vi "Recipe example.vi"() -> ()   [LabVIEW 2020, in "SMCD14_lib.lvlib"]
uses:
  SMCD14_lib.lvlib
  Macro Cluster.ctl
  typedefAxisConfiguration.ctl
panel:
  in  "Actiomn":u16(ring) items=["NONE", "Start", "Stop", "Clear", "Motor ON", "Motor OFF"]
  in  "Move type:-NoCalib":u16(ring) items=["Absolute"=1, "Relative"=2, "Velocity"=3, "none"=0]
  in  "Move type:-Full":u16(ring) items=["Absolute"=1, "Relative"=2, "Velocity"=3, "Homing"=4, "none"=0]
  out "AllowCalib":bool
  in  "Recipe":i32(listbox)
  in  "Macro Cluster":T1={"Macro Type"=0, "Macro Name"="", "Macro Description"="", "M1_action_axis 1"=0, "M1_action_axis 2"=0, "M1_action_axis 3"=0, "M1_action_axis 4"=0, "M1_action_axis 5"=0, "M1_action_axis 6"=0, "M2_Axis"=0, "M2_Target_Pos"=0.0, "M2_Target_Vel"=0.0, "MoveModeControl"=0, "M3_1_Time"=0, "M3_Type"=0, "M3_2_wait_for_axis 1"=FALSE, "M3_2_wait_for_axis 2"=FALSE, "M3_2_wait_for_axis 3"=FALSE, "M3_2_wait_for_axis 4"=FALSE, "M3_2_wait_for_axis 5"=FALSE, "M3_2_wait_for_axis 6"=FALSE, "M3_3_mesage"="", "M3_3_wait_for_calib"=FALSE, "SelectedTargetCtrl"=1, "M5_select_action"=0} caption="Cluster 2" {"M5_select_action" items=["Stop", "Safe Position", "Working Position", "Run scaning", "Transfer posituin"]; "SelectedTargetCtrl" items=["none", "Target 1", "Target 2", "Target 3", "Target 4", "Target 5", "Target 6", "Laser test"]; "M3_Type" items=["Type1", "Type2", "Type3", "Type4", "Type5"]; "M3_1_Time" format="%<%H:%M:%S>t"; "MoveModeControl" items=["Absolute"=1, "Relative"=2, "Velocity"=3, "Homing"=4, "none"=0]; "M2_Target_Vel" format="%<%H:%M:%S>t"; "M2_Axis" items=["Axis no1", "Axis no2", "Axis no3", "Axis no4", "Axis no5", "Axis no6"]; "M1_action_axis 6" items=["NONE", "Start", "Stop", "Clear", "Motor ON", "motor OFF"]; "M1_action_axis 5" items=["NONE", "Start", "Stop", "Clear", "Motor ON", "motor OFF"]; "M1_action_axis 4" items=["NONE", "Start", "Stop", "Clear", "Motor ON", "motor OFF"]; "M1_action_axis 3" items=["------", "Manual", "Time SP", "Thickness SP"]; "M1_action_axis 2" items=["NONE", "Start", "Stop", "Clear", "Motor ON", "motor OFF"]; "M1_action_axis 1" items=["NONE", "Start", "Stop", "Clear", "Motor ON", "motor OFF"]; "Macro Type" items=["Action", "Parameters", "Wait"]}
  in  "Macro to add:":u16(ring) items=["Action", "Parameters", "Wait"]
  in  "Remove":bool
  in  "Add":bool
  in  "Next":bool
  in  "Back":bool
  out "AxisaMaxSpeed":dbl[](array[numeric])
  out "AxisaMinSpeed":dbl[](array[numeric])
  in  "AxisConfigurations":T2[](array[typedef]) {"AxisMaxSpeed" format="%#_6f"; "AxisMinSpeed" format="%#_6f"; "UnitsControl" items=["mm", "°"]}
  out "edit?":bool
  in  "Open Button":bool
  in  "Save Button":bool
  in  "New Button":bool
  in  "Macro Description:":string
  in  "Macro name:":string
  in  "Macro:":u16(ring) items=["Action", "Parameters", "Wait"]
  in  "Tab Control":enum32{"M1", "M2", "M3"}(tab)
  in  "Axis 1 action:":u16(ring) caption="Axis 1 axis action:" items=["NONE", "Start", "Stop", "Clear", "Motor ON", "Motor OFF"]
  in  "Axis 2 action:":u16(ring) caption="Axis 2 axis action:" items=["NONE", "Start", "Stop", "Clear", "Motor ON", "Motor OFF"]
  in  "Axis 3 action:":u16(ring) caption="Axis 2 axis action:" items=["NONE", "Start", "Stop", "Clear", "Motor ON", "Motor OFF"]
  in  "Axis 4 action:":u16(ring) caption="Axis 4 axis action:" items=["NONE", "Start", "Stop", "Clear", "Motor ON", "Motor OFF"]
  in  "Axis 5 action:":u16(ring) caption="Axis 5 axis action:" items=["NONE", "Start", "Stop", "Clear", "Motor ON", "Motor OFF"]
  in  "Axis 6 action:":u16(ring) caption="Axis 6 axis action:" items=["NONE", "Start", "Stop", "Clear", "Motor ON", "Motor OFF"]
  in  "Act. Step":i32
  in  "Axis:":u16(ring)
  in  "Target pos.:":sgl format="%#_6f unit"
  in  "Target vel.:":sgl caption="Wait Time" format="%#_6f unit/s"
  in  "Move type:":u16(ring) caption="Energy voltage SP:" items=["Absolute"=1, "Relative"=2, "Velocity"=3, "none"=0]
  in  "M3_Type":u16(ring) items=["Wait for time", "wait for axis", "wait for user action"]
  in  "Tab -Wait":enum32{"1", "2", "3"}(tab)
  in  "Time:":u32 caption="Shutter Time SP:" format="%<%H:%M:%S>t"
  out "Remaining\ntime:":i32 caption="Shutter Time SP:" format="%<%H:%M:%S>t"
  in  "wait for Homed":bool
  in  "wait for axis 1":bool
  in  "wait for axis 2":bool
  in  "wait for axis 3":bool
  in  "wait for axis 4":bool
  in  "wait for axis 5":bool
  in  "wait for axis 6":bool
  in  "Mesage:":string
  out "AxisNames":string[](array[string])
  in  "Current Macro":T1={"Macro Type"=0, "Macro Name"="", "Macro Description"="", "M1_action_axis 1"=0, "M1_action_axis 2"=0, "M1_action_axis 3"=0, "M1_action_axis 4"=0, "M1_action_axis 5"=0, "M1_action_axis 6"=0, "M2_Axis"=0, "M2_Target_Pos"=0.0, "M2_Target_Vel"=0.0, "MoveModeControl"=0, "M3_1_Time"=0, "M3_Type"=0, "M3_2_wait_for_axis 1"=FALSE, "M3_2_wait_for_axis 2"=FALSE, "M3_2_wait_for_axis 3"=FALSE, "M3_2_wait_for_axis 4"=FALSE, "M3_2_wait_for_axis 5"=FALSE, "M3_2_wait_for_axis 6"=FALSE, "M3_3_mesage"="", "M3_3_wait_for_calib"=FALSE, "SelectedTargetCtrl"=1, "M5_select_action"=0} caption="Cluster 2" {"M5_select_action" items=["Stop", "Safe Position", "Working Position", "Run scaning", "Transfer posituin"]; "SelectedTargetCtrl" items=["none", "Target 1", "Target 2", "Target 3", "Target 4", "Target 5", "Target 6", "Laser test"]; "M3_Type" items=["Type1", "Type2", "Type3", "Type4", "Type5"]; "M3_1_Time" format="%<%H:%M:%S>t"; "MoveModeControl" items=["Absolute"=1, "Relative"=2, "Velocity"=3, "Homing"=4, "none"=0]; "M2_Target_Vel" format="%<%H:%M:%S>t"; "M2_Axis" items=["Axis no1", "Axis no2", "Axis no3", "Axis no4", "Axis no5", "Axis no6"]; "M1_action_axis 6" items=["NONE", "Start", "Stop", "Clear", "Motor ON", "motor OFF"]; "M1_action_axis 5" items=["NONE", "Start", "Stop", "Clear", "Motor ON", "motor OFF"]; "M1_action_axis 4" items=["NONE", "Start", "Stop", "Clear", "Motor ON", "motor OFF"]; "M1_action_axis 3" items=["------", "Manual", "Time SP", "Thickness SP"]; "M1_action_axis 2" items=["NONE", "Start", "Stop", "Clear", "Motor ON", "motor OFF"]; "M1_action_axis 1" items=["NONE", "Start", "Stop", "Clear", "Motor ON", "motor OFF"]; "Macro Type" items=["Action", "Parameters", "Wait"]}
  in  "Macro Table":T1[](array[typedef]) {"M5_select_action" items=["Stop", "Safe Position", "Working Position", "Run scaning", "Transfer posituin"]; "SelectedTargetCtrl" items=["none", "Target 1", "Target 2", "Target 3", "Target 4", "Target 5", "Target 6", "Laser test"]; "M3_Type" items=["Type1", "Type2", "Type3", "Type4", "Type5"]; "M3_1_Time" format="%<%H:%M:%S>t"; "MoveModeControl" items=["Absolute"=1, "Relative"=2, "Velocity"=3, "Homing"=4, "none"=0]; "M2_Target_Vel" format="%<%H:%M:%S>t"; "M2_Axis" items=["Axis no1", "Axis no2", "Axis no3", "Axis no4", "Axis no5", "Axis no6"]; "M1_action_axis 6" items=["NONE", "Start", "Stop", "Clear", "Motor ON", "motor OFF"]; "M1_action_axis 5" items=["NONE", "Start", "Stop", "Clear", "Motor ON", "motor OFF"]; "M1_action_axis 4" items=["NONE", "Start", "Stop", "Clear", "Motor ON", "motor OFF"]; "M1_action_axis 3" items=["------", "Manual", "Time SP", "Thickness SP"]; "M1_action_axis 2" items=["NONE", "Start", "Stop", "Clear", "Motor ON", "motor OFF"]; "M1_action_axis 1" items=["NONE", "Start", "Stop", "Clear", "Motor ON", "motor OFF"]; "Macro Type" items=["Action", "Parameters", "Wait"]}
  out "size":i32
  # "Przykładowy silnik do zaawansowanych receptur w LabView\nw zależności od wybranego typu ukruwane/ pokazywane są \npola do edycji.\nw liście Recipe pokazywany jest podląd wszystkich receptur, \nmożna kliknąć w wybraną - okno Macro przełączy sie na wybraną\nnawigować moża przyciskami <-- i -->\nmożda dodać kolejne makro lub usunąc aktywne"
  # "Lista makr:\nx- SET data:\nx    Power SP\nx    Voltage SP\nx    Current SP\n\nx- SET shutter data\nx    Working mode - Manual nie dostępny\nx    Thicknes SP\nx    Time SP\n\nx- SET MFC setpoint\nx    Flow SP\n\nx- SET Operate/Standby\nx- Open/Close Shutter\nx- Open/Close MFC\n- Wait for Time\n    Time \n- wait for close Shutter"
  # "Select action for each axes:"
  # "Set axis parameters:"
  # "Select wait mode:"
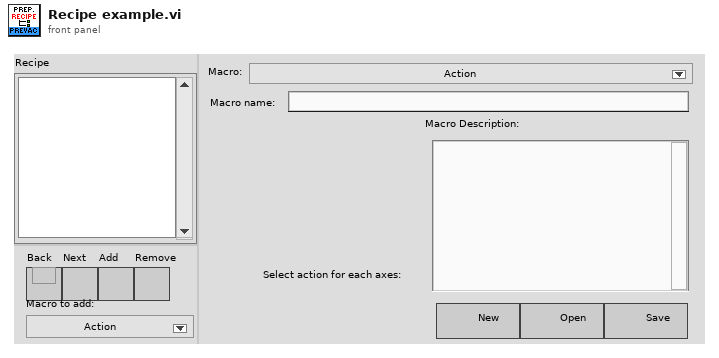
[diagram p1: front panel]
types:
  T1 = typedef "SMCD14_lib.lvlib/Macro Cluster.ctl" = cluster{"Macro Type":u16, "Macro Name":string, "Macro Description":string, "M1_action_axis 1":u16, "M1_action_axis 2":u16, "M1_action_axis 3":u16, "M1_action_axis 4":u16, "M1_action_axis 5":u16, "M1_action_axis 6":u16, "M2_Axis":u16, "M2_Target_Pos":sgl, "M2_Target_Vel":sgl, "MoveModeControl":u16, "M3_1_Time":u32, "M3_Type":u16, "M3_2_wait_for_axis 1":bool, "M3_2_wait_for_axis 2":bool, "M3_2_wait_for_axis 3":bool, "M3_2_wait_for_axis 4":bool, "M3_2_wait_for_axis 5":bool, "M3_2_wait_for_axis 6":bool, "M3_3_mesage":string, "M3_3_wait_for_calib":bool, "SelectedTargetCtrl":u16, "M5_select_action":u16}
  T2 = typedef "SMCD14_lib.lvlib/typedefAxisConfiguration.ctl" = cluster{"AxisName":string, "UnitsControl":u16, "AxisSlaveID":u16, "AxisBaseAddr":u16, "AxisMinSpeed":dbl, "AxisMaxSpeed":dbl}
  T3 = enum16{"open", "replace", "create", "open or create", "replace or create", "replace or create with confirmation"}
  T4 = typedef "LVStringsAndValuesArrayTypeDef_U16.ctl" = cluster{"String":string, "Value":u16}[]
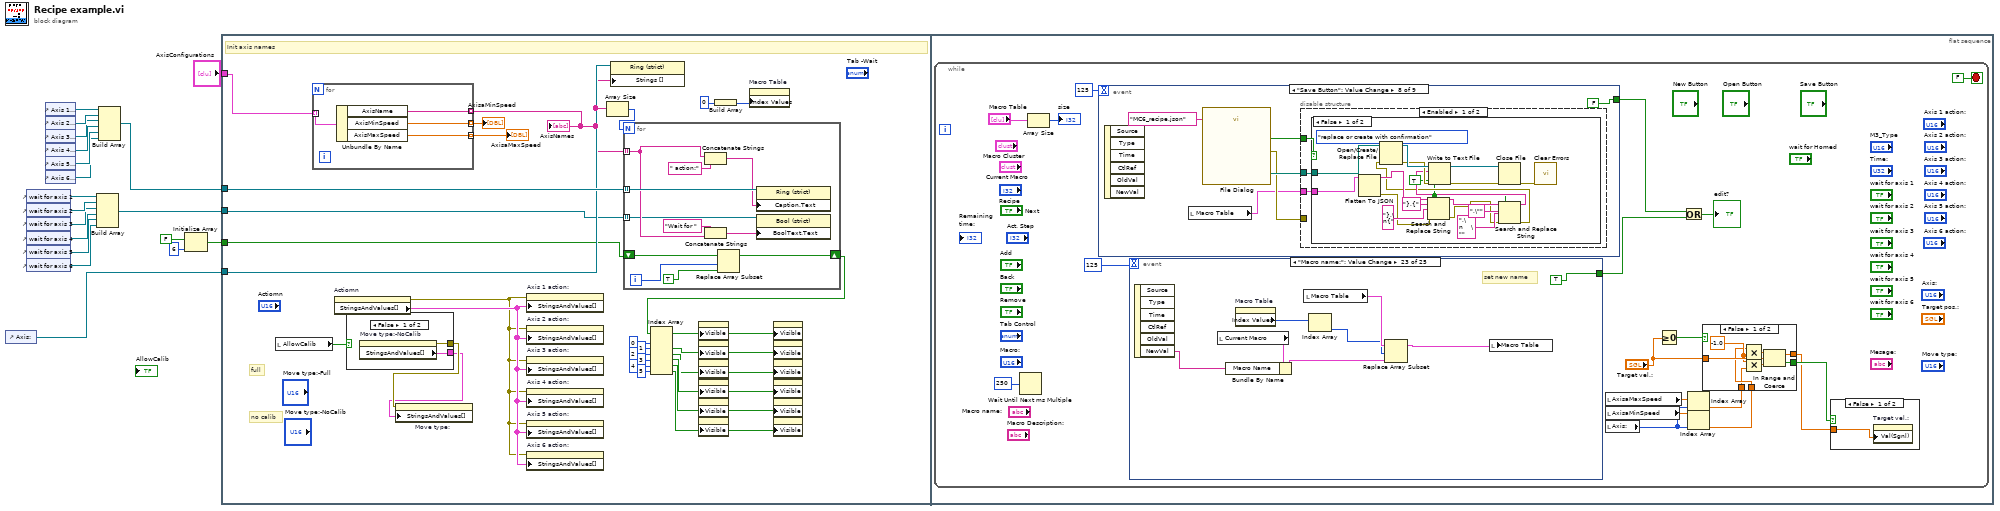
[diagram p0: block diagram]
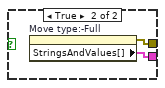
[diagram p2: hidden frame]
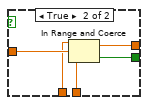
[diagram p4: hidden frame]
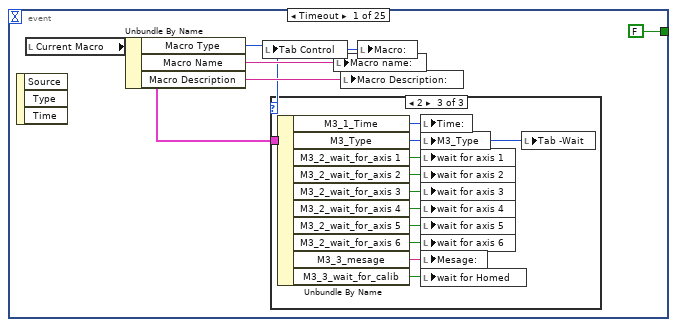
[diagram p5: hidden frame]
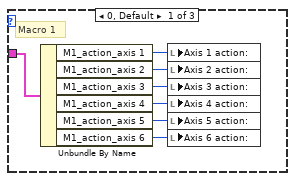
[diagram p6: hidden frame]
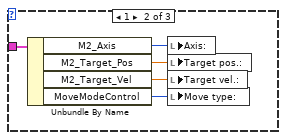
[diagram p7: hidden frame]
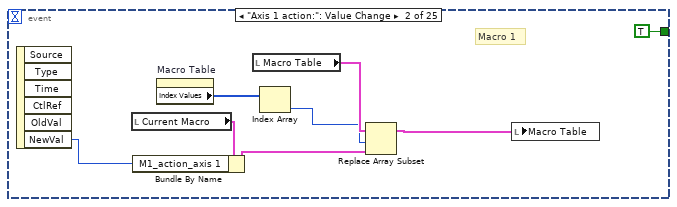
[diagram p8: hidden frame]
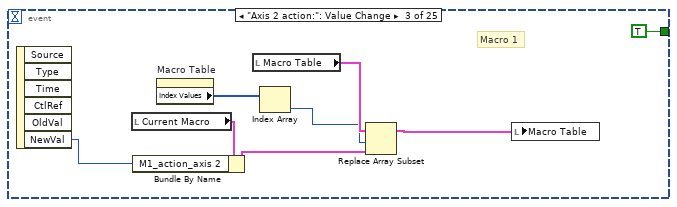
[diagram p9: hidden frame]
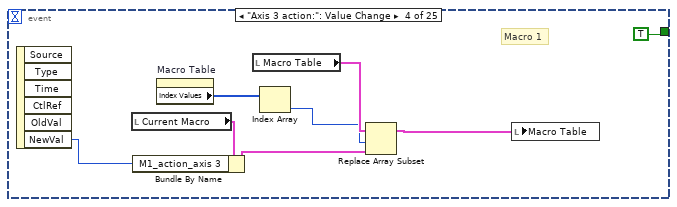
[diagram p10: hidden frame]
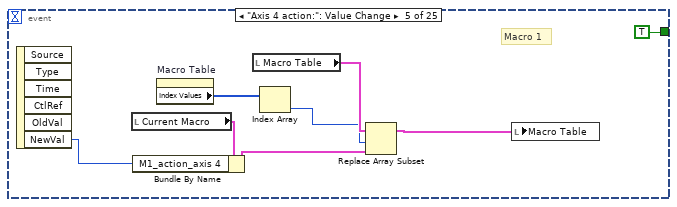
[diagram p11: hidden frame]
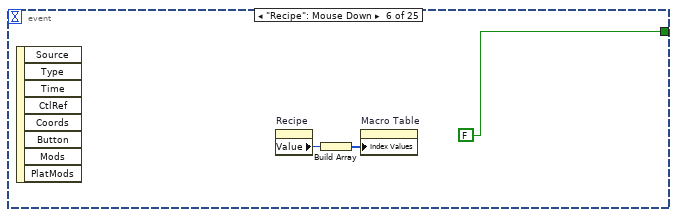
[diagram p12: hidden frame]
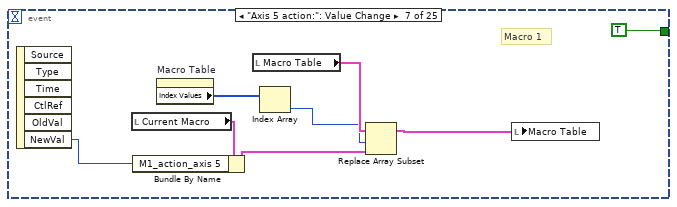
[diagram p13: hidden frame]
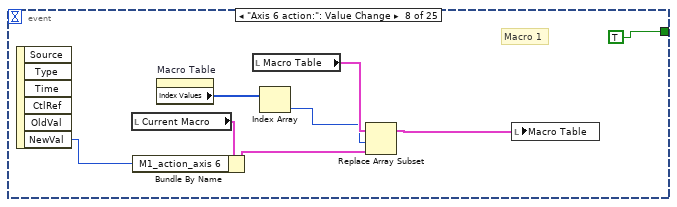
[diagram p14: hidden frame]
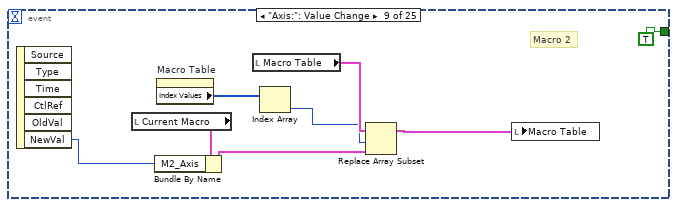
[diagram p15: hidden frame]
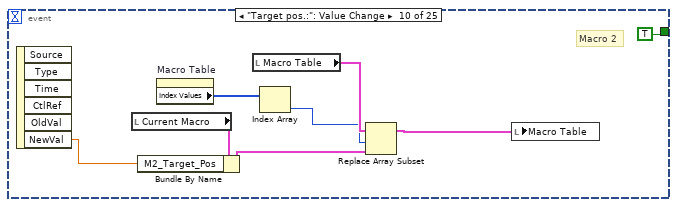
[diagram p16: hidden frame]
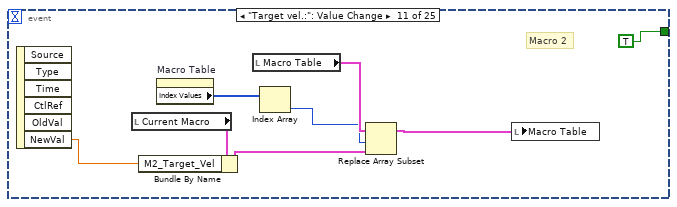
[diagram p17: hidden frame]
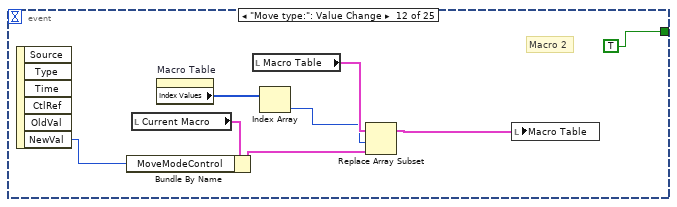
[diagram p18: hidden frame]
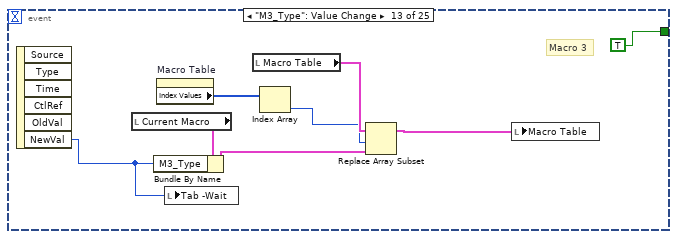
[diagram p19: hidden frame]
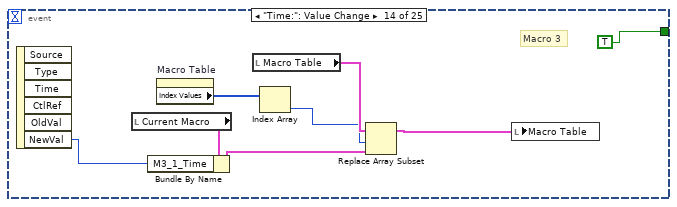
[diagram p20: hidden frame]
diagram:
  n1 = control-ref of="Axis:"() -> (w12:refnum<vi>)
  n2 = control-ref of="wait for axis 1"() -> (w11:refnum<vi>)
  n3 = control-ref of="wait for axis 2"() -> (w10:refnum<vi>)
  n4 = control-ref of="wait for axis 3"() -> (w9:refnum<vi>)
  n5 = control-ref of="wait for axis 4"() -> (w6:refnum<vi>)
  n6 = control-ref of="wait for axis 5"() -> (w8:refnum<vi>)
  n7 = control-ref of="wait for axis 6"() -> (w7:refnum<vi>)
  n8 = control-ref of="Axis 1 action:"() -> (w19:refnum<vi>)
  n9 = control-ref of="Axis 2 action:"() -> (w14:refnum<vi>)
  n10 = control-ref of="Axis 3 action:"() -> (w13:refnum<vi>)
  n11 = control-ref of="Axis 4 action:"() -> (w18:refnum<vi>)
  n12 = control-ref of="Axis 5 action:"() -> (w17:refnum<vi>)
  n13 = control-ref of="Axis 6 action:"() -> (w16:refnum<vi>)
  n14 = Build Array(w11, w10, w9, w6, w8, w7) -> (w5:refnum<vi>[])
  n15 = Build Array(w19, w14, w13, w18, w17, w16) -> (w15:refnum<vi>[])
  n16 = Initialize Array(FALSE, 6 ("dimension size")) -> (w1:bool[])
  n17 = flat-sequence {
    tunnel: w15 -> [w48]
    tunnel: w12 -> [w47]
    tunnel: w5 -> [w46]
    tunnel: "AxisConfigurations" -> [w44]
    tunnel: w1 -> [w36]
    frame #0 {
      # "no calib"
      # "full"
      # "Init axis names"
      n18 = local read "AllowCalib"() -> (w41:bool)
      n19 = for {
        tunnel: w44 -> [w56] mode=indexing
        tunnel: [w55] -> w28 mode=indexing
        tunnel: [w54] -> w43 mode=indexing
        tunnel: [w53] -> w42 mode=indexing
        n20 = Unbundle By Name(w56) -> ("AxisName"=w55:string, "AxisMinSpeed"=w54:dbl, "AxisMaxSpeed"=w53:dbl)
      }
      "AxisNames" <- w28
      "AxisaMinSpeed" <- w43
      "AxisaMaxSpeed" <- w42
      n21 = property on="Actiomn" class="Ring (strict)"() -> (error out=w39:errorcluster, "StringsAndValues[]"=w40:T4)  [unwired: 2 in, 1 out]
      n22 = case shown="False" w41 {
        tunnel: [w50 w51] -> w37
        tunnel: [w49 w52] -> w38
        frame False {
          n23 = property on="Move type:-NoCalib" class="Ring (strict)"() -> (error out=w49:errorcluster, "StringsAndValues[]"=w50:T4)  [unwired: 2 in, 1 out]
        }
        frame True {
          n24 = property on="Move type:-Full" class="Ring (strict)"() -> (error out=w52:errorcluster, "StringsAndValues[]"=w51:T4)  [unwired: 2 in, 1 out]
        }
      }
      n25 = property on="Move type:" class="Ring (strict)"(error in=w38, "StringsAndValues[]"=w37) -> ()  [unwired: 1 in, 2 out]
      n26 = property on="Axis 1 action:" class="Ring (strict)"(error in=w39, "StringsAndValues[]"=w40) -> ()  [unwired: 1 in, 2 out]
      n27 = property on="Axis 2 action:" class="Ring (strict)"(error in=w39, "StringsAndValues[]"=w40) -> ()  [unwired: 1 in, 2 out]
      n28 = property on="Axis 3 action:" class="Ring (strict)"(error in=w39, "StringsAndValues[]"=w40) -> ()  [unwired: 1 in, 2 out]
      n29 = property on="Axis 4 action:" class="Ring (strict)"(error in=w39, "StringsAndValues[]"=w40) -> ()  [unwired: 1 in, 2 out]
      n30 = property on="Axis 5 action:" class="Ring (strict)"(error in=w39, "StringsAndValues[]"=w40) -> ()  [unwired: 1 in, 2 out]
      n31 = property on="Axis 6 action:" class="Ring (strict)"(error in=w39, "StringsAndValues[]"=w40) -> ()  [unwired: 1 in, 2 out]
      n32 = Array Size(array=w28) -> (size(s)=w27:i32)
      n33 = property class="Ring (strict)"(reference=w47, "Strings []"=w28) -> ()  [unwired: 1 in, 2 out]
      n34 = for {
        N: w27 -> [_]
        tunnel: w28 -> [w63] mode=indexing
        tunnel: w48 -> [w66] mode=indexing
        tunnel: w46 -> [w61] mode=indexing
        shift-right: [w57] -> w29
        shift-left: w36 -> [w60]
        i -> [w59]
        n35 = Concatenate Strings(w63, " action:" ("Label.Text")) -> (w65:string)
        n36 = Concatenate Strings("Wait for " ("Label.Text"), w63) -> (w62:string)
        n37 = Replace Array Subset(array=w60, new element=TRUE, index=w59) -> (w57:bool[])
        n38 = property class="Ring (strict)"(reference=w66, "Caption.Text"=w65) -> ()  [unwired: 1 in, 2 out]
        n39 = property class="Bool (strict)"(reference=w61, "BoolText.Text"=w62) -> ()  [unwired: 1 in, 2 out]
      }
      n40 = Index Array(array=w29, index #1=0 ("dimension size"), index #2=1 ("dimension size"), index #3=2 ("dimension size"), index #4=3 ("dimension size"), index #5=4 ("dimension size"), index #6=5 ("dimension size")) -> (element #1=w26:bool, element #2=w25:bool, element #3=w21:bool, element #4=w24:bool, element #5=w23:bool, element #6=w22:bool)
      n41 = property on="Axis 1 action:" class="Ring (strict)"("Visible"=w26) -> ()  [unwired: 2 in, 2 out]
      n42 = property on="Axis 2 action:" class="Ring (strict)"("Visible"=w25) -> ()  [unwired: 2 in, 2 out]
      n43 = property on="Axis 3 action:" class="Ring (strict)"("Visible"=w21) -> ()  [unwired: 2 in, 2 out]
      n44 = property on="Axis 4 action:" class="Ring (strict)"("Visible"=w24) -> ()  [unwired: 2 in, 2 out]
      n45 = property on="Axis 5 action:" class="Ring (strict)"("Visible"=w23) -> ()  [unwired: 2 in, 2 out]
      n46 = property on="Axis 6 action:" class="Ring (strict)"("Visible"=w22) -> ()  [unwired: 2 in, 2 out]
      n47 = Build Array(0) -> (w20:i32[])
      n48 = property on="Macro Table" class="Arr (strict)"("Index Values"=w20) -> ()  [unwired: 2 in, 2 out]
      n49 = property on="wait for axis 1" class="Bool (strict)"("Visible"=w26) -> ()  [unwired: 2 in, 2 out]
      n50 = property on="wait for axis 2" class="Bool (strict)"("Visible"=w25) -> ()  [unwired: 2 in, 2 out]
      n51 = property on="wait for axis 3" class="Bool (strict)"("Visible"=w21) -> ()  [unwired: 2 in, 2 out]
      n52 = property on="wait for axis 4" class="Bool (strict)"("Visible"=w24) -> ()  [unwired: 2 in, 2 out]
      n53 = property on="wait for axis 5" class="Bool (strict)"("Visible"=w23) -> ()  [unwired: 2 in, 2 out]
      n54 = property on="wait for axis 6" class="Bool (strict)"("Visible"=w22) -> ()  [unwired: 2 in, 2 out]
    }
    frame #1 {
      n55 = while {
        stop <- FALSE ("stop") stop-if-true
        n56 = Wait Until Next ms Multiple(millisecond multiple=u32 250) -> ()  [unwired: 1 out]
        n57 = Array Size(array="Macro Table") -> (size(s)=→"size":i32)
        n58 = event shown="[7] \"Save Button\": Value Change" {
          selector: _ -> [_ _ _ _ _ _ _ _ _]
          dyn-events: _ -> [_ _ _ _ _ _ _ _ _]
          timeout: 125 -> [_ _ _ _ _ _ _ _ _]
          tunnel: [FALSE FALSE FALSE FALSE TRUE TRUE TRUE FALSE TRUE] -> w79
          event Timeout {
            n59 = event-data() -> ()  [unwired: 1 in, 3 out]
            n60 = local read "Macro Table"() -> (w319:T1[])
            n61 = property on="Macro Table" class="Arr (strict)"() -> ("Index Values"=w321:u32[])  [unwired: 2 in, 2 out]
            n62 = for {
              tunnel: w319 -> [w333] mode=indexing
              tunnel: [w329] -> w317 mode=indexing
              tunnel: [w322] -> w316 mode=indexing
              i -> [w325]
              n63 = local read "Act. Step"() -> (w324:i32)
              n64 = Unbundle By Name(w333) -> ("Macro Type"=w331:u16, "Macro Name"=w326:string)
              n65 = property on="Macro to add:" class="Ring (strict)"() -> ("Strings []"=w332:string[])  [unwired: 2 in, 2 out]
              n66 = Subtract(x=w325, y=w324) -> (x-y=w323:i32)
              n67 = Index Array(array=w332, index=w331) -> (element=w330:string)
              n68 = case shown="..-1, Default" w323 {
                tunnel: [1 4 0] -> w322
                frame ..-1, Default {
                }
                frame 0 {
                }
                frame 1.. {
                }
              }
              n69 = Concatenate Strings(w330, "\r", "   | ", w326) -> (w329:string)
            }
            n70 = Index Array(array=w321) -> (element=w320:u32)  [unwired: 1 in]
            n71 = local write "Recipe"(w320) -> ()
            n72 = Index Array(array=w319, index=w320) -> (element=w318:T1)
            n73 = local write "Current Macro"(w318) -> ()
            n74 = property on="Recipe" class="LstBox (strict)"("Item Names"=w317) -> ()  [unwired: 2 in, 2 out]
            n75 = property on="Recipe" class="LstBox (strict)"("Item Symbols"=w316) -> ()  [unwired: 2 in, 2 out]
          }
          event Panel Close {
            n76 = event-data() -> ()  [unwired: 1 in, 4 out]
            n77 = Stop(stop? (T)=TRUE) -> ()
          }
          event "Next": Value Change {
            n78 = event-data() -> ()  [unwired: 1 in, 6 out]
            n79 = property on="Macro Table" class="Arr (strict)"() -> ("Index Values"=w340:u32[])  [unwired: 2 in, 2 out]
            n80 = local read "size"() -> (w345:i32)
            n81 = Index Array(array=w340) -> (element=w343:u32)  [unwired: 1 in]
            n82 = Decrement(x=w345) -> (x-1=w344:i32)
            n83 = Increment(x=w343) -> (x+1=w346:u32)
            n84 = In Range and Coerce(upper limit=w344, x=w346, lower limit=i16 0) -> (coerced(x)=w342:u32)  [unwired: 1 out]
            n85 = Build Array(w342) -> (w341:u32[])
            n86 = property on="Macro Table" class="Arr (strict)"("Index Values"=w341) -> ()  [unwired: 2 in, 2 out]
          }
          event "Back": Value Change {
            n87 = event-data() -> ()  [unwired: 1 in, 6 out]
            n88 = property on="Macro Table" class="Arr (strict)"() -> ("Index Values"=w352:u32[])  [unwired: 2 in, 2 out]
            n89 = Index Array(array=w352) -> (element=w351:u32)  [unwired: 1 in]
            n90 = Less Or Equal To 0?(x=w351) -> (x <= 0?=w353:bool)
            n91 = case shown="False" w353 {
              tunnel: w351 -> [w355 w356]
              tunnel: [w354 w356] -> w350
              frame False {
                n92 = Decrement(x=w355) -> (x-1=w354:u32)
              }
              frame True {
              }
            }
            n93 = Build Array(w350) -> (w349:u32[])
            n94 = property on="Macro Table" class="Arr (strict)"("Index Values"=w349) -> ()  [unwired: 2 in, 2 out]
          }
          event "Remove": Value Change {
            n95 = event-data() -> ()  [unwired: 1 in, 6 out]
            n96 = local read "size"() -> (w358:i32)
            n97 = property on="Macro Table" class="Arr (strict)"() -> ("Index Values"=w362:u32[])  [unwired: 2 in, 2 out]
            n98 = Index Array(array=w362) -> (element=w361:u32)  [unwired: 1 in]
            n99 = Greater?(x=w358, y=u32 1) -> (0:w359:bool)
            n100 = case shown="True" w359 {
              tunnel: w361 -> [_ w365]
              frame False {
              }
              frame True {
                n101 = local read "Macro Table"() -> (w367:T1[])
                n102 = Decrement(x=w365) -> (x-1=w364:u32)
                n103 = Delete From Array(array=w367, index=w365) -> (array with subset deleted=w366:T1[])  [unwired: 1 in, 1 out]
                n104 = local write "Macro Table"(w366) -> ()
                n105 = Build Array(w364) -> (w363:u32[])
                n106 = property on="Macro Table" class="Arr (strict)"("Index Values"=w363) -> ()  [unwired: 2 in, 2 out]
              }
            }
          }
          event "Add": Value Change {
            n107 = event-data() -> ()  [unwired: 1 in, 6 out]
            n108 = property on="Macro Table" class="Arr (strict)"() -> ("Index Values"=w377:u32[])  [unwired: 2 in, 2 out]
            n109 = local read "Macro Cluster"() -> (w370:T1)
            n110 = local read "Macro Table"() -> (w375:T1[])
            n111 = Bundle By Name(cluster=w370, "Macro Type"="Macro to add:") -> (w369:T1)
            n112 = Index Array(array=w377) -> (element=w374:u32)  [unwired: 1 in]
            n113 = Increment(x=w374) -> (x+1=w372:u32)
            n114 = Insert Into Array(array=w375, index=w372, new element=w369) -> (w373:T1[])
            n115 = Build Array(w372) -> (w376:u32[])
            n116 = local write "Macro Table"(w373) -> ()
            n117 = property on="Macro Table" class="Arr (strict)"("Index Values"=w376) -> ()  [unwired: 2 in, 2 out]
          }
          event "New Button": Value Change {
            n118 = event-data() -> ()  [unwired: 1 in, 6 out]
            n119 = Build Array(0) -> (w380:i32[])
            n120 = property on="Macro Table" class="Arr (strict)"("Index Values"=w380) -> ()  [unwired: 2 in, 2 out]
            n121 = local write "Macro Table"(T1[] [{"Macro Type"=0, "Macro Name"="", "Macro Description"="", "M1_action_axis 1"=0, "M1_action_axis 2"=0, "M1_action_axis 3"=0, "M1_action_axis 4"=0, "M1_action_axis 5"=0, "M1_action_axis 6"=0, "M2_Axis"=0, "M2_Target_Pos"=0.0, "M2_Target_Vel"=0.0, "MoveModeControl"=0, "M3_1_Time"=0, "M3_Type"=0, "M3_2_wait_for_axis 1"=FALSE, "M3_2_wait_for_axis 2"=FALSE, "M3_2_wait_for_axis 3"=FALSE, "M3_2_wait_for_axis 4"=FALSE, "M3_2_wait_for_axis 5"=FALSE, "M3_2_wait_for_axis 6"=FALSE, "M3_3_mesage"="", "M3_3_wait_for_calib"=FALSE, "SelectedTargetCtrl"=1, "M5_select_action"=0}] ("Macro Table")) -> ()
          }
          event "Save Button": Value Change {
            n122 = event-data() -> ()  [unwired: 1 in, 6 out]
            n123 = local read "Macro Table"() -> (w382:T1[])
            n124 = call "File Dialog"("default name"="MC6_recipe.json") -> ("selected path"=w385:path, "cancelled"=w386:bool, "error out"=w383:errorcluster)  [unwired: 11 in, 1 out]
            n125 = disable-structure shown="Enabled" {
              disable-tunnel: w386 -> [w390 w413]
              disable-tunnel: w385 -> [w389 w412]
              disable-tunnel: w382 -> [w388 w411]
              disable-tunnel: w383 -> [_ w410]
              frame Enabled {
                n126 = case shown="False" w390 {
                  tunnel: w389 -> [w409 _]
                  tunnel: w388 -> [w402 _]
                  frame False {
                    w391 = TRUE ("replace all? (F)")
                    n127 = Flatten To JSON(anything=w402) -> (JSON string=w398:string, 11:w399:errorcluster)  [unwired: 2 in]
                    n128 = Search and Replace String(replace all?=w391, input string=w398, search string="},{", replace string="},\n{" ("search string"), error in=w399) -> (result string=w397:string, error out=w393:errorcluster)  [unwired: 3 in, 2 out]
                    n129 = Search and Replace String(replace all?=w391, input string=w397, search string=",\"", replace string=",\n    \"" ("search string"), error in=w393) -> (result string=w394:string, error out=w392:errorcluster)  [unwired: 3 in, 2 out]
                    n130 = Open/Create/Replace File(file path (use dialog)=w409, error in=w392, operation (0:open)=T3."replace or create with confirmation") -> (refnum out=w407:refnum<file>, error out=w406:errorcluster)  [unwired: 3 in, 1 out]
                    n131 = Write to Text File(file (use dialog)=w407, text=w394, error in=w406) -> (refnum out=w405:refnum<file>, error out=w404:errorcluster)  [unwired: 1 in, 1 out]
                    n132 = Close File(refnum=w405, error in=w404) -> (error out=w403:errorcluster)  [unwired: 1 out]
                    n133 = call <vilib>:"Clear Errors.vi"("error in (no error)"=w403) -> ()  [unwired: 5 in, 2 out]
                  }
                  frame True {
                  }
                }
              }
              frame Disabled {
                n134 = case shown="False" w413 {
                  tunnel: w412 -> [w423 _]
                  tunnel: w411 -> [w416 _]
                  tunnel: w410 -> [w415 _]
                  frame False {
                    (unwired) TRUE ("replace all? (F)")
                    n135 = Flatten To XML(6:w416) -> (2:w414:string)
                    n136 = Open/Create/Replace File(file path (use dialog)=w423, error in=w415, operation (0:open)=T3."replace or create with confirmation") -> (refnum out=w421:refnum<file>, error out=w420:errorcluster)  [unwired: 3 in, 1 out]
                    n137 = Write to Text File(file (use dialog)=w421, text=w414, error in=w420) -> (refnum out=w419:refnum<file>, error out=w418:errorcluster)  [unwired: 1 in, 1 out]
                    n138 = Close File(refnum=w419, error in=w418) -> (error out=w417:errorcluster)  [unwired: 1 out]
                    n139 = call <vilib>:"Clear Errors.vi"("error in (no error)"=w417) -> ()  [unwired: 5 in, 2 out]
                  }
                  frame True {
                  }
                }
              }
            }
          }
          event "Open Button": Value Change {
            n140 = event-data() -> ()  [unwired: 1 in, 6 out]
            n141 = local read "Macro Table"() -> (w427:T1[])
            n142 = call "File Dialog2"("default name"="MC6_recipe.json") -> ("selected path"=w429:path, "exists"=w428:bool, "cancelled"=w430:bool)  [unwired: 11 in, 1 out]
            n143 = case shown="False" w430 {
              tunnel: w429 -> [w435 _]
              tunnel: w428 -> [w433 _]
              tunnel: w427 -> [w434 _]
              tunnel: [w432 0] -> w425
              frame False {
                n144 = disable-structure shown="Enabled" {
                  disable-tunnel: w435 -> [w439 w452]
                  disable-tunnel: w434 -> [w438 w451]
                  disable-tunnel: w433 -> [w437 w453]
                  disable-tunnel: [0 _] -> w432
                  frame Enabled {
                    n145 = case shown="True" w437 {
                      tunnel: w439 -> [_ w450]
                      tunnel: w438 -> [_ w444]
                      frame False {
                      }
                      frame True {
                        n146 = Open/Create/Replace File(file path (use dialog)=w450, operation (0:open)=T3."open") -> (refnum out=w447:refnum<file>, error out=w446:errorcluster)  [unwired: 4 in, 1 out]
                        n147 = Read from Text File(file (use dialog)=w447, error in=w446) -> (refnum out=w440:refnum<file>, text=w445:string, error out=w441:errorcluster)  [unwired: 2 in, 1 out]
                        n148 = Unflatten From JSON(JSON string=w445, type and defaults=w444, error in (no error)=w441) -> (value=w443:T1[], error out=w442:errorcluster)  [unwired: 4 in]
                        n149 = Close File(refnum=w440, error in=w442) -> (error out=w448:errorcluster)  [unwired: 1 out]
                        n150 = local write "Macro Table"(w443) -> ()
                        n151 = call <vilib>:"Clear Errors.vi"("error in (no error)"=w448) -> ()  [unwired: 5 in, 2 out]
                      }
                    }
                  }
                  frame Disabled {
                    n152 = case shown="True" w453 {
                      tunnel: w452 -> [_ w464]
                      tunnel: w451 -> [_ w458]
                      frame False {
                      }
                      frame True {
                        n153 = Open/Create/Replace File(file path (use dialog)=w464, operation (0:open)=T3."open") -> (refnum out=w461:refnum<file>, error out=w460:errorcluster)  [unwired: 4 in, 1 out]
                        n154 = Read from Text File(file (use dialog)=w461, error in=w460) -> (refnum out=w459:refnum<file>, text=w457:string, error out=w456:errorcluster)  [unwired: 2 in, 1 out]
                        n155 = Unflatten From XML(xml string=w457, type=w458, error in (no error)=w456) -> (value=w455:T1[], error out=w454:errorcluster)
                        n156 = Close File(refnum=w459, error in=w454) -> (error out=w462:errorcluster)  [unwired: 1 out]
                        n157 = local write "Macro Table"(w455) -> ()
                        n158 = call <vilib>:"Clear Errors.vi"("error in (no error)"=w462) -> ()  [unwired: 5 in, 2 out]
                      }
                    }
                  }
                }
              }
              frame True {
              }
            }
            n159 = Build Array(w425) -> (w426:i32[])
            n160 = property on="Macro Table" class="Arr (strict)"("Index Values"=w426) -> ()  [unwired: 2 in, 2 out]
          }
        }
        n161 = event shown="[22] \"Macro name:\": Value Change" {
          selector: _ -> [_ _ _ _ _ _ _ _ _ _ _ _ _ _ _ _ _ _ _ _ _ _ _ _ _]
          dyn-events: _ -> [_ _ _ _ _ _ _ _ _ _ _ _ _ _ _ _ _ _ _ _ _ _ _ _ _]
          timeout: 125 -> [_ _ _ _ _ _ _ _ _ _ _ _ _ _ _ _ _ _ _ _ _ _ _ _ _]
          tunnel: [FALSE TRUE TRUE TRUE TRUE FALSE TRUE TRUE TRUE TRUE TRUE TRUE TRUE TRUE TRUE TRUE TRUE TRUE TRUE TRUE TRUE TRUE TRUE TRUE TRUE] -> w78
          event Timeout {
            n162 = event-data() -> ()  [unwired: 1 in, 3 out]
            n163 = local read "Current Macro"() -> (w102:T1)
            n164 = Unbundle By Name(w102) -> ("Macro Type"=w101:u16, "Macro Name"=w104:string, "Macro Description"=w103:string)
            n165 = local write "Tab Control"(w101) -> ()
            n166 = case shown="2" w101 {
              tunnel: w102 -> [w111 w116 w127]
              frame 0, Default {
                # "Macro 1"
                n167 = Unbundle By Name(w111) -> ("M1_action_axis 1"=w110:u16, "M1_action_axis 2"=w109:u16, "M1_action_axis 3"=w108:u16, "M1_action_axis 4"=w107:u16, "M1_action_axis 5"=w106:u16, "M1_action_axis 6"=w105:u16)
                n168 = local write "Axis 1 action:"(w110) -> ()
                n169 = local write "Axis 2 action:"(w109) -> ()
                n170 = local write "Axis 3 action:"(w108) -> ()
                n171 = local write "Axis 4 action:"(w107) -> ()
                n172 = local write "Axis 5 action:"(w106) -> ()
                n173 = local write "Axis 6 action:"(w105) -> ()
              }
              frame 1 {
                n174 = Unbundle By Name(w116) -> ("M2_Axis"=w115:u16, "M2_Target_Pos"=w114:sgl, "M2_Target_Vel"=w113:sgl, "MoveModeControl"=w112:u16)
                n175 = local write "Axis:"(w115) -> ()
                n176 = local write "Target pos.:"(w114) -> ()
                n177 = local write "Target vel.:"(w113) -> ()
                n178 = local write "Move type:"(w112) -> ()
              }
              frame 2 {
                n179 = Unbundle By Name(w127) -> ("M3_1_Time"=w126:u32, "M3_Type"=w118:u16, "M3_2_wait_for_axis 1"=w125:bool, "M3_2_wait_for_axis 2"=w124:bool, "M3_2_wait_for_axis 3"=w123:bool, "M3_2_wait_for_axis 4"=w122:bool, "M3_2_wait_for_axis 5"=w121:bool, "M3_2_wait_for_axis 6"=w120:bool, "M3_3_mesage"=w119:string, "M3_3_wait_for_calib"=w117:bool)
                n180 = local write "Time:"(w126) -> ()
                n181 = local write "M3_Type"(w118) -> ()
                n182 = local write "wait for axis 1"(w125) -> ()
                n183 = local write "wait for axis 2"(w124) -> ()
                n184 = local write "wait for axis 3"(w123) -> ()
                n185 = local write "wait for axis 4"(w122) -> ()
                n186 = local write "wait for axis 5"(w121) -> ()
                n187 = local write "wait for axis 6"(w120) -> ()
                n188 = local write "Mesage:"(w119) -> ()
                n189 = local write "wait for Homed"(w117) -> ()
                n190 = local write "Tab -Wait"(w118) -> ()
              }
            }
            n191 = local write "Macro name:"(w104) -> ()
            n192 = local write "Macro Description:"(w103) -> ()
            n193 = local write "Macro:"(w101) -> ()
          }
          event "Axis 1 action:": Value Change {
            # "Macro 1"
            n194 = event-data() -> ("NewVal"=w129:u16)  [unwired: 1 in, 5 out]
            n195 = local read "Current Macro"() -> (w135:T1)
            n196 = Bundle By Name(cluster=w135, "M1_action_axis 1"=w129) -> (w134:T1)
            n197 = property on="Macro Table" class="Arr (strict)"() -> ("Index Values"=w133:u32[])  [unwired: 2 in, 2 out]
            n198 = local read "Macro Table"() -> (w131:T1[])
            n199 = Index Array(array=w133) -> (element=w130:u32)  [unwired: 1 in]
            n200 = Replace Array Subset(array=w131, new element=w134, index=w130) -> (w132:T1[])
            n201 = local write "Macro Table"(w132) -> ()
          }
          event "Axis 2 action:": Value Change {
            # "Macro 1"
            n202 = event-data() -> ("NewVal"=w137:u16)  [unwired: 1 in, 5 out]
            n203 = local read "Current Macro"() -> (w143:T1)
            n204 = Bundle By Name(cluster=w143, "M1_action_axis 2"=w137) -> (w142:T1)
            n205 = property on="Macro Table" class="Arr (strict)"() -> ("Index Values"=w141:u32[])  [unwired: 2 in, 2 out]
            n206 = local read "Macro Table"() -> (w139:T1[])
            n207 = Index Array(array=w141) -> (element=w138:u32)  [unwired: 1 in]
            n208 = Replace Array Subset(array=w139, new element=w142, index=w138) -> (w140:T1[])
            n209 = local write "Macro Table"(w140) -> ()
          }
          event "Axis 3 action:": Value Change {
            # "Macro 1"
            n210 = event-data() -> ("NewVal"=w145:u16)  [unwired: 1 in, 5 out]
            n211 = local read "Current Macro"() -> (w151:T1)
            n212 = Bundle By Name(cluster=w151, "M1_action_axis 3"=w145) -> (w150:T1)
            n213 = property on="Macro Table" class="Arr (strict)"() -> ("Index Values"=w149:u32[])  [unwired: 2 in, 2 out]
            n214 = local read "Macro Table"() -> (w147:T1[])
            n215 = Index Array(array=w149) -> (element=w146:u32)  [unwired: 1 in]
            n216 = Replace Array Subset(array=w147, new element=w150, index=w146) -> (w148:T1[])
            n217 = local write "Macro Table"(w148) -> ()
          }
          event "Axis 4 action:": Value Change {
            # "Macro 1"
            n218 = event-data() -> ("NewVal"=w153:u16)  [unwired: 1 in, 5 out]
            n219 = local read "Current Macro"() -> (w159:T1)
            n220 = Bundle By Name(cluster=w159, "M1_action_axis 4"=w153) -> (w158:T1)
            n221 = property on="Macro Table" class="Arr (strict)"() -> ("Index Values"=w157:u32[])  [unwired: 2 in, 2 out]
            n222 = local read "Macro Table"() -> (w155:T1[])
            n223 = Index Array(array=w157) -> (element=w154:u32)  [unwired: 1 in]
            n224 = Replace Array Subset(array=w155, new element=w158, index=w154) -> (w156:T1[])
            n225 = local write "Macro Table"(w156) -> ()
          }
          event "Recipe": Mouse Down {
            n226 = event-data() -> ()  [unwired: 1 in, 8 out]
            n227 = property on="Recipe" class="LstBox (strict)"() -> ("Value"=w161:i32)  [unwired: 2 in, 2 out]
            n228 = Build Array(w161) -> (w162:i32[])
            n229 = property on="Macro Table" class="Arr (strict)"("Index Values"=w162) -> ()  [unwired: 2 in, 2 out]
          }
          event "Axis 5 action:": Value Change {
            # "Macro 1"
            n230 = event-data() -> ("NewVal"=w164:u16)  [unwired: 1 in, 5 out]
            n231 = local read "Current Macro"() -> (w170:T1)
            n232 = Bundle By Name(cluster=w170, "M1_action_axis 5"=w164) -> (w169:T1)
            n233 = property on="Macro Table" class="Arr (strict)"() -> ("Index Values"=w168:u32[])  [unwired: 2 in, 2 out]
            n234 = local read "Macro Table"() -> (w166:T1[])
            n235 = Index Array(array=w168) -> (element=w165:u32)  [unwired: 1 in]
            n236 = Replace Array Subset(array=w166, new element=w169, index=w165) -> (w167:T1[])
            n237 = local write "Macro Table"(w167) -> ()
          }
          event "Axis 6 action:": Value Change {
            # "Macro 1"
            n238 = event-data() -> ("NewVal"=w172:u16)  [unwired: 1 in, 5 out]
            n239 = local read "Current Macro"() -> (w178:T1)
            n240 = Bundle By Name(cluster=w178, "M1_action_axis 6"=w172) -> (w177:T1)
            n241 = property on="Macro Table" class="Arr (strict)"() -> ("Index Values"=w176:u32[])  [unwired: 2 in, 2 out]
            n242 = local read "Macro Table"() -> (w174:T1[])
            n243 = Index Array(array=w176) -> (element=w173:u32)  [unwired: 1 in]
            n244 = Replace Array Subset(array=w174, new element=w177, index=w173) -> (w175:T1[])
            n245 = local write "Macro Table"(w175) -> ()
          }
          event "Axis:": Value Change {
            # "Macro 2"
            n246 = event-data() -> ("NewVal"=w180:u16)  [unwired: 1 in, 5 out]
            n247 = local read "Current Macro"() -> (w186:T1)
            n248 = Bundle By Name(cluster=w186, "M2_Axis"=w180) -> (w185:T1)
            n249 = property on="Macro Table" class="Arr (strict)"() -> ("Index Values"=w184:u32[])  [unwired: 2 in, 2 out]
            n250 = local read "Macro Table"() -> (w182:T1[])
            n251 = Index Array(array=w184) -> (element=w181:u32)  [unwired: 1 in]
            n252 = Replace Array Subset(array=w182, new element=w185, index=w181) -> (w183:T1[])
            n253 = local write "Macro Table"(w183) -> ()
          }
          event "Target pos.:": Value Change {
            # "Macro 2"
            n254 = event-data() -> ("NewVal"=w188:sgl)  [unwired: 1 in, 5 out]
            n255 = local read "Current Macro"() -> (w194:T1)
            n256 = Bundle By Name(cluster=w194, "M2_Target_Pos"=w188) -> (w193:T1)
            n257 = property on="Macro Table" class="Arr (strict)"() -> ("Index Values"=w192:u32[])  [unwired: 2 in, 2 out]
            n258 = local read "Macro Table"() -> (w190:T1[])
            n259 = Index Array(array=w192) -> (element=w189:u32)  [unwired: 1 in]
            n260 = Replace Array Subset(array=w190, new element=w193, index=w189) -> (w191:T1[])
            n261 = local write "Macro Table"(w191) -> ()
          }
          event "Target vel.:": Value Change {
            # "Macro 2"
            n262 = event-data() -> ("NewVal"=w196:sgl)  [unwired: 1 in, 5 out]
            n263 = local read "Current Macro"() -> (w202:T1)
            n264 = Bundle By Name(cluster=w202, "M2_Target_Vel"=w196) -> (w201:T1)
            n265 = property on="Macro Table" class="Arr (strict)"() -> ("Index Values"=w200:u32[])  [unwired: 2 in, 2 out]
            n266 = local read "Macro Table"() -> (w198:T1[])
            n267 = Index Array(array=w200) -> (element=w197:u32)  [unwired: 1 in]
            n268 = Replace Array Subset(array=w198, new element=w201, index=w197) -> (w199:T1[])
            n269 = local write "Macro Table"(w199) -> ()
          }
          event "Move type:": Value Change {
            # "Macro 2"
            n270 = event-data() -> ("NewVal"=w204:u16)  [unwired: 1 in, 5 out]
            n271 = local read "Current Macro"() -> (w210:T1)
            n272 = Bundle By Name(cluster=w210, "MoveModeControl"=w204) -> (w209:T1)
            n273 = property on="Macro Table" class="Arr (strict)"() -> ("Index Values"=w208:u32[])  [unwired: 2 in, 2 out]
            n274 = local read "Macro Table"() -> (w206:T1[])
            n275 = Index Array(array=w208) -> (element=w205:u32)  [unwired: 1 in]
            n276 = Replace Array Subset(array=w206, new element=w209, index=w205) -> (w207:T1[])
            n277 = local write "Macro Table"(w207) -> ()
          }
          event "M3_Type": Value Change {
            # "Macro 3"
            n278 = event-data() -> ("NewVal"=w212:u16)  [unwired: 1 in, 5 out]
            n279 = local read "Current Macro"() -> (w218:T1)
            n280 = Bundle By Name(cluster=w218, "M3_Type"=w212) -> (w217:T1)
            n281 = property on="Macro Table" class="Arr (strict)"() -> ("Index Values"=w216:u32[])  [unwired: 2 in, 2 out]
            n282 = local write "Tab -Wait"(w212) -> ()
            n283 = local read "Macro Table"() -> (w214:T1[])
            n284 = Index Array(array=w216) -> (element=w213:u32)  [unwired: 1 in]
            n285 = Replace Array Subset(array=w214, new element=w217, index=w213) -> (w215:T1[])
            n286 = local write "Macro Table"(w215) -> ()
          }
          event "Time:": Value Change {
            # "Macro 3"
            n287 = event-data() -> ("NewVal"=w220:u32)  [unwired: 1 in, 5 out]
            n288 = local read "Current Macro"() -> (w226:T1)
            n289 = Bundle By Name(cluster=w226, "M3_1_Time"=w220) -> (w225:T1)
            n290 = property on="Macro Table" class="Arr (strict)"() -> ("Index Values"=w224:u32[])  [unwired: 2 in, 2 out]
            n291 = local read "Macro Table"() -> (w222:T1[])
            n292 = Index Array(array=w224) -> (element=w221:u32)  [unwired: 1 in]
            n293 = Replace Array Subset(array=w222, new element=w225, index=w221) -> (w223:T1[])
            n294 = local write "Macro Table"(w223) -> ()
          }
          event "wait for axis 1": Value Change {
            # "Macro 3"
            n295 = event-data() -> ("NewVal"=w228:bool)  [unwired: 1 in, 5 out]
            n296 = local read "Current Macro"() -> (w234:T1)
            n297 = Bundle By Name(cluster=w234, "M3_2_wait_for_axis 1"=w228) -> (w233:T1)
            n298 = property on="Macro Table" class="Arr (strict)"() -> ("Index Values"=w232:u32[])  [unwired: 2 in, 2 out]
            n299 = local read "Macro Table"() -> (w230:T1[])
            n300 = Index Array(array=w232) -> (element=w229:u32)  [unwired: 1 in]
            n301 = Replace Array Subset(array=w230, new element=w233, index=w229) -> (w231:T1[])
            n302 = local write "Macro Table"(w231) -> ()
          }
          event "wait for axis 2": Value Change {
            # "Macro 3"
            n303 = event-data() -> ("NewVal"=w236:bool)  [unwired: 1 in, 5 out]
            n304 = local read "Current Macro"() -> (w242:T1)
            n305 = Bundle By Name(cluster=w242, "M3_2_wait_for_axis 2"=w236) -> (w241:T1)
            n306 = property on="Macro Table" class="Arr (strict)"() -> ("Index Values"=w240:u32[])  [unwired: 2 in, 2 out]
            n307 = local read "Macro Table"() -> (w238:T1[])
            n308 = Index Array(array=w240) -> (element=w237:u32)  [unwired: 1 in]
            n309 = Replace Array Subset(array=w238, new element=w241, index=w237) -> (w239:T1[])
            n310 = local write "Macro Table"(w239) -> ()
          }
          event "wait for axis 3": Value Change {
            # "Macro 3"
            n311 = event-data() -> ("NewVal"=w244:bool)  [unwired: 1 in, 5 out]
            n312 = local read "Current Macro"() -> (w250:T1)
            n313 = Bundle By Name(cluster=w250, "M3_2_wait_for_axis 3"=w244) -> (w249:T1)
            n314 = property on="Macro Table" class="Arr (strict)"() -> ("Index Values"=w248:u32[])  [unwired: 2 in, 2 out]
            n315 = local read "Macro Table"() -> (w246:T1[])
            n316 = Index Array(array=w248) -> (element=w245:u32)  [unwired: 1 in]
            n317 = Replace Array Subset(array=w246, new element=w249, index=w245) -> (w247:T1[])
            n318 = local write "Macro Table"(w247) -> ()
          }
          event "wait for axis 4": Value Change {
            # "Macro 3"
            n319 = event-data() -> ("NewVal"=w252:bool)  [unwired: 1 in, 5 out]
            n320 = local read "Current Macro"() -> (w258:T1)
            n321 = Bundle By Name(cluster=w258, "M3_2_wait_for_axis 4"=w252) -> (w257:T1)
            n322 = property on="Macro Table" class="Arr (strict)"() -> ("Index Values"=w256:u32[])  [unwired: 2 in, 2 out]
            n323 = local read "Macro Table"() -> (w254:T1[])
            n324 = Index Array(array=w256) -> (element=w253:u32)  [unwired: 1 in]
            n325 = Replace Array Subset(array=w254, new element=w257, index=w253) -> (w255:T1[])
            n326 = local write "Macro Table"(w255) -> ()
          }
          event "wait for axis 5": Value Change {
            # "Macro 3"
            n327 = event-data() -> ("NewVal"=w260:bool)  [unwired: 1 in, 5 out]
            n328 = local read "Current Macro"() -> (w266:T1)
            n329 = Bundle By Name(cluster=w266, "M3_2_wait_for_axis 5"=w260) -> (w265:T1)
            n330 = property on="Macro Table" class="Arr (strict)"() -> ("Index Values"=w264:u32[])  [unwired: 2 in, 2 out]
            n331 = local read "Macro Table"() -> (w262:T1[])
            n332 = Index Array(array=w264) -> (element=w261:u32)  [unwired: 1 in]
            n333 = Replace Array Subset(array=w262, new element=w265, index=w261) -> (w263:T1[])
            n334 = local write "Macro Table"(w263) -> ()
          }
          event "wait for axis 6": Value Change {
            # "Macro 3"
            n335 = event-data() -> ("NewVal"=w268:bool)  [unwired: 1 in, 5 out]
            n336 = local read "Current Macro"() -> (w274:T1)
            n337 = Bundle By Name(cluster=w274, "M3_2_wait_for_axis 6"=w268) -> (w273:T1)
            n338 = property on="Macro Table" class="Arr (strict)"() -> ("Index Values"=w272:u32[])  [unwired: 2 in, 2 out]
            n339 = local read "Macro Table"() -> (w270:T1[])
            n340 = Index Array(array=w272) -> (element=w269:u32)  [unwired: 1 in]
            n341 = Replace Array Subset(array=w270, new element=w273, index=w269) -> (w271:T1[])
            n342 = local write "Macro Table"(w271) -> ()
          }
          event "wait for Homed": Value Change {
            # "Macro 3"
            n343 = event-data() -> ("NewVal"=w276:bool)  [unwired: 1 in, 5 out]
            n344 = local read "Current Macro"() -> (w282:T1)
            n345 = Bundle By Name(cluster=w282, "M3_3_wait_for_calib"=w276) -> (w281:T1)
            n346 = property on="Macro Table" class="Arr (strict)"() -> ("Index Values"=w280:u32[])  [unwired: 2 in, 2 out]
            n347 = local read "Macro Table"() -> (w278:T1[])
            n348 = Index Array(array=w280) -> (element=w277:u32)  [unwired: 1 in]
            n349 = Replace Array Subset(array=w278, new element=w281, index=w277) -> (w279:T1[])
            n350 = local write "Macro Table"(w279) -> ()
          }
          event "Mesage:": Value Change {
            # "Macro 3"
            n351 = event-data() -> ("NewVal"=w284:string)  [unwired: 1 in, 5 out]
            n352 = local read "Current Macro"() -> (w290:T1)
            n353 = Bundle By Name(cluster=w290, "M3_3_mesage"=w284) -> (w289:T1)
            n354 = property on="Macro Table" class="Arr (strict)"() -> ("Index Values"=w288:u32[])  [unwired: 2 in, 2 out]
            n355 = local read "Macro Table"() -> (w286:T1[])
            n356 = Index Array(array=w288) -> (element=w285:u32)  [unwired: 1 in]
            n357 = Replace Array Subset(array=w286, new element=w289, index=w285) -> (w287:T1[])
            n358 = local write "Macro Table"(w287) -> ()
          }
          event "Macro name:": Value Change {
            # "set new name"
            n359 = event-data() -> ("NewVal"=w293:string)  [unwired: 1 in, 5 out]
            n360 = local read "Current Macro"() -> (w298:T1)
            n361 = Bundle By Name(cluster=w298, "Macro Name"=w293) -> (w297:T1)
            n362 = property on="Macro Table" class="Arr (strict)"() -> ("Index Values"=w291:u32[])  [unwired: 2 in, 2 out]
            n363 = local read "Macro Table"() -> (w295:T1[])
            n364 = Index Array(array=w291) -> (element=w294:u32)  [unwired: 1 in]
            n365 = Replace Array Subset(array=w295, new element=w297, index=w294) -> (w296:T1[])
            n366 = local write "Macro Table"(w296) -> ()
          }
          event "Macro Description:": Value Change {
            # "set new name"
            n367 = event-data() -> ("NewVal"=w300:string)  [unwired: 1 in, 5 out]
            n368 = local read "Current Macro"() -> (w306:T1)
            n369 = Bundle By Name(cluster=w306, "Macro Description"=w300) -> (w305:T1)
            n370 = property on="Macro Table" class="Arr (strict)"() -> ("Index Values"=w304:u32[])  [unwired: 2 in, 2 out]
            n371 = local read "Macro Table"() -> (w302:T1[])
            n372 = Index Array(array=w304) -> (element=w301:u32)  [unwired: 1 in]
            n373 = Replace Array Subset(array=w302, new element=w305, index=w301) -> (w303:T1[])
            n374 = local write "Macro Table"(w303) -> ()
          }
          event "Macro:": Value Change {
            n375 = event-data() -> ("NewVal"=w313:u16)  [unwired: 1 in, 5 out]
            n376 = local read "Current Macro"() -> (w314:T1)
            n377 = Bundle By Name(cluster=w314, "Macro Type"=w313) -> (w312:T1)
            n378 = property on="Macro Table" class="Arr (strict)"() -> ("Index Values"=w311:u32[])  [unwired: 2 in, 2 out]
            n379 = local read "Macro Table"() -> (w309:T1[])
            n380 = Index Array(array=w311) -> (element=w308:u32)  [unwired: 1 in]
            n381 = Replace Array Subset(array=w309, new element=w312, index=w308) -> (w310:T1[])
            n382 = local write "Macro Table"(w310) -> ()
          }
        }
        n383 = local read "AxisaMaxSpeed"() -> (w76:dbl[])
        n384 = local read "AxisaMinSpeed"() -> (w75:dbl[])
        n385 = local read "Axis:"() -> (w74:u16)
        n386 = Greater Or Equal To 0?(x="Target vel.:") -> (x >= 0?=w73:bool)
        n387 = Or(x=w79, y=w78) -> (x .or. y?=→"edit?":bool)
        n388 = Index Array(array=w76, index=w74) -> (element=w71:dbl)
        n389 = Index Array(array=w75, index=w74) -> (element=w70:dbl)
        n390 = case shown="False" w73 {
          tunnel: "Target vel.:" -> [w94 w99]
          tunnel: w71 -> [w87 w98]
          tunnel: w70 -> [w88 w97]
          tunnel: [w93 w96] -> w68
          tunnel: [w92 w95] -> w69
          frame False {
            w89 = -1.0 ("x")
            n391 = Multiply(x=w88, y=w89) -> (x*y=w91:dbl)
            n392 = Multiply(x=w89, y=w87) -> (x*y=w90:dbl)
            n393 = In Range and Coerce(upper limit=w91, x=w94, lower limit=w90) -> (coerced(x)=w93:dbl, In Range?=w92:bool)
          }
          frame True {
            n394 = In Range and Coerce(upper limit=w98, x=w99, lower limit=w97) -> (coerced(x)=w96:dbl, In Range?=w95:bool)
          }
        }
        n395 = case shown="False" w69 {
          tunnel: w68 -> [w86 _]
          frame False {
            n396 = property on="Target vel.:" class="DigNum (strict)"("Val(Sgnl)"=w86) -> ()  [unwired: 2 in, 2 out]
          }
          frame True {
          }
        }
      }
    }
  }
